vi "pid-tuning.vi"() -> ()   [LabVIEW 2019]
uses:
  <vilib>/DAQmx/read.llb/DAQmx Read (Analog 1D DBL 1Chan NSamp).vi
  <vilib>/Analysis/baseanly.llb/Mean (DBL).vi
  <vilib>/DAQmx/write.llb/DAQmx Write (Analog DBL 1Chan 1Samp).vi
  <vilib>/DAQmx/create/channels.llb/DAQmx Create Channel (AO-Current-Basic).vi
  <vilib>/DAQmx/create/channels.llb/DAQmx Create Channel (AI-Current-Basic).vi
  <vilib>/DAQmx/miscellaneous.llb/DAQmx Fill In Error Info.vi
  <vilib>/addons/control/pid/pid.llb/PID (DBL).vi
  <vilib>/Analysis/NI_AALBase.lvlib
  <vilib>/addons/control/pid/NI_PID_pid.lvlib
panel:
  out "PID FINAL POWER":dbl
  in  "stop":bool
  out "PID START TIME":dbl
  in  "Tabs":T1(tab)
  in  "POWER CONTROL":dbl format="%#_13g"
  in  "ENABLE FURNACE TEST":bool[](array[boolean])=[FALSE]
  in  "STOP FURNACE TEST":bool[](array[boolean])=[FALSE]
  out "PYROMETER READING":dbl
  in  "RAMP UP POWER":dbl format="%#_13g"
  out "TEMPERATURE OVER TIME":cluster{dbl[], dbl[]}[](graph)
  out "CURRENT TEMPERATURE (C)":dbl
  in  "PID SETPOINT":dbl=820.0
  in  "Clear Data":bool
  in  "Restart PID":bool
  in  "PID gains":T2={"proportional gain (Kc)"=5e-05, "integral time (Ti, min)"=1.5, "derivative time (Td, min)"=0.0} {"derivative time (Td, min)" format="%.8f"; "integral time (Ti, min)" format="%.24f"; "proportional gain (Kc)" format="%.8f"}
  out "POWER LEVEL OUTPUT (%)":dbl
  in  "Time Target (s)":dbl=1.0
  in  "Auto Ramp":bool
  out "Current setpoint":dbl
  in  "Max temp":dbl
  out "Time has Elapsed 2":bool caption="Time has Elapsed"
  out "CURRENT RAMP DOWN POWER LEVEL":string
  out "PYROMETER READING 2":dbl
  in  "RAMP DOWN TIME (min)":dbl=10.0
  in  "Mode":T3(ring)
  out "PYROMETER TEMP":dbl
  in  "POWER OUT":dbl format="%#_13g"
  in  "STOP FURNACE":bool[](array[boolean])
  in  "ENABLE FURNACE":bool[](array[boolean])
  out "DONE":bool
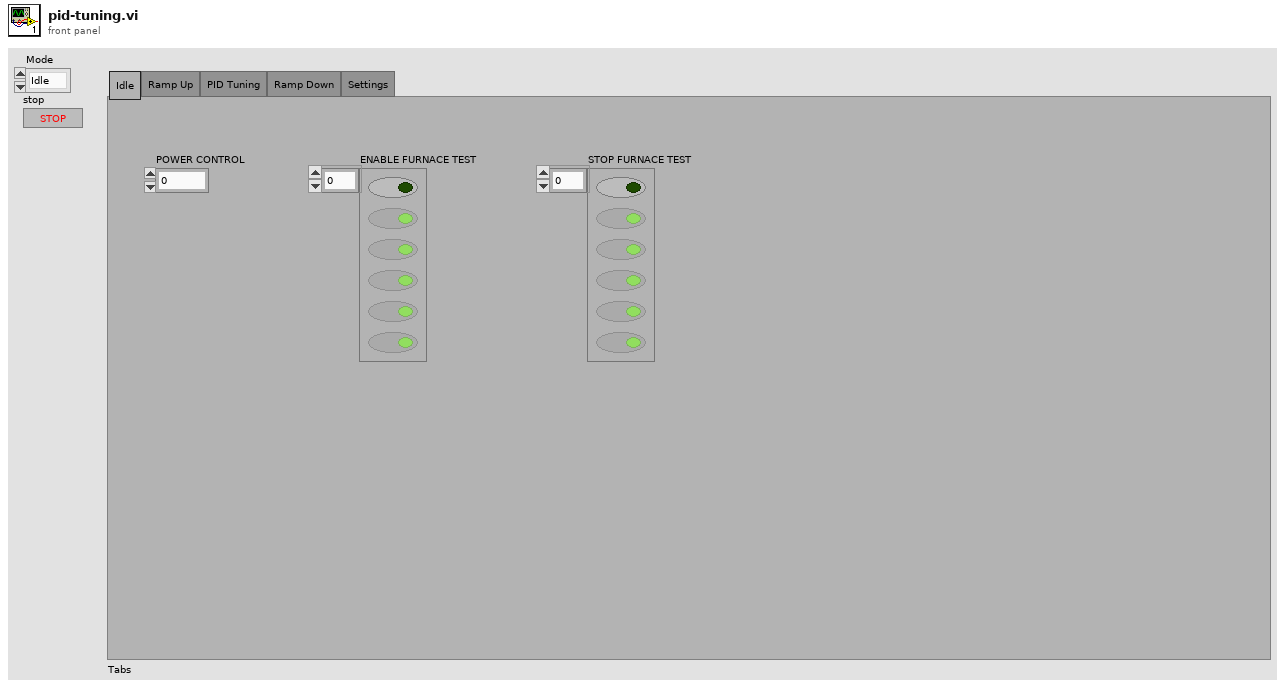
[diagram p1: front panel]
types:
  T1 = enum32{"Idle", "Ramp Up", "PID Tuning", "Ramp Down", "Settings"}
  T2 = cluster{"proportional gain (Kc)":dbl, "integral time (Ti, min)":dbl, "derivative time (Td, min)":dbl}
  T3 = enum16{"Idle", "Ramp Up", "PID Tune", "Ramp Down"}
  T4 = enum8{"Enabled", "Disabled", "Disabled and Grayed Out"}
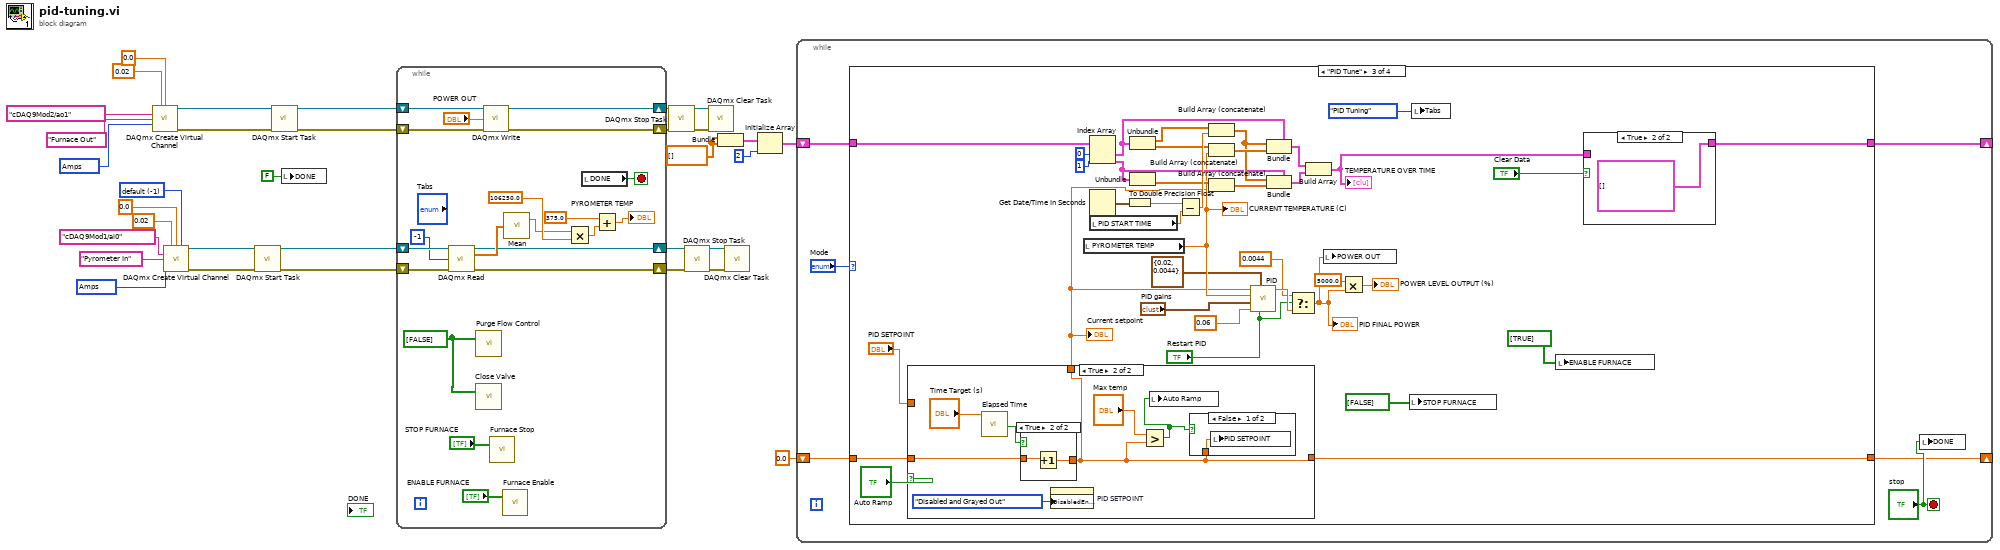
[diagram p0: block diagram]
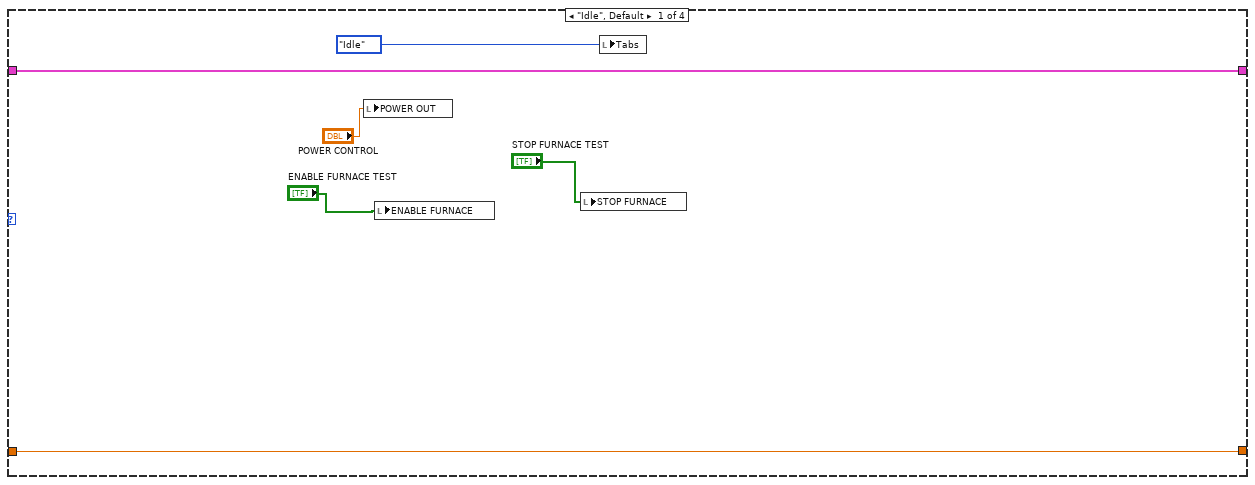
[diagram p2: hidden frame]
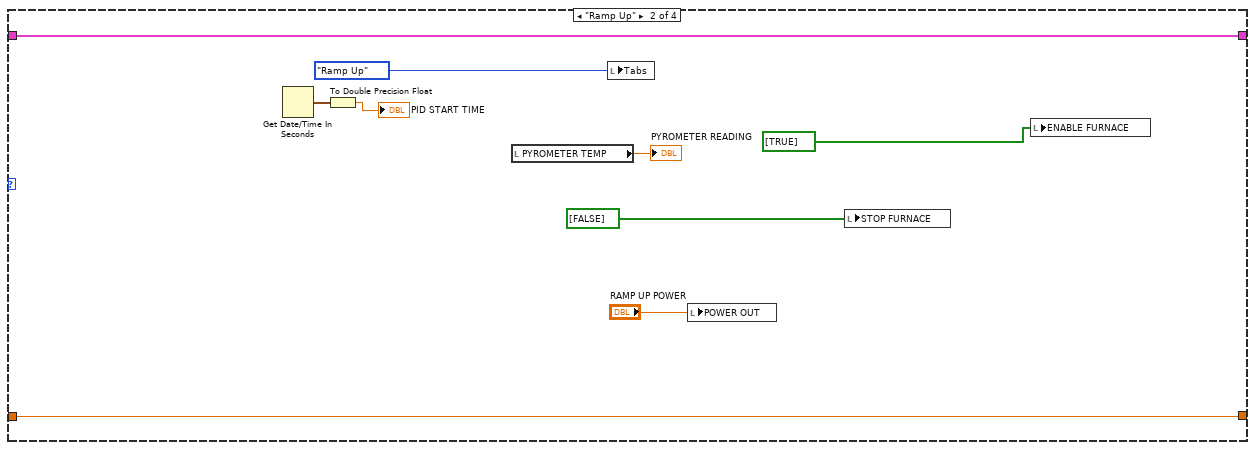
[diagram p3: hidden frame]
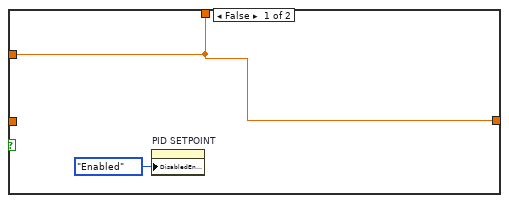
[diagram p4: hidden frame]
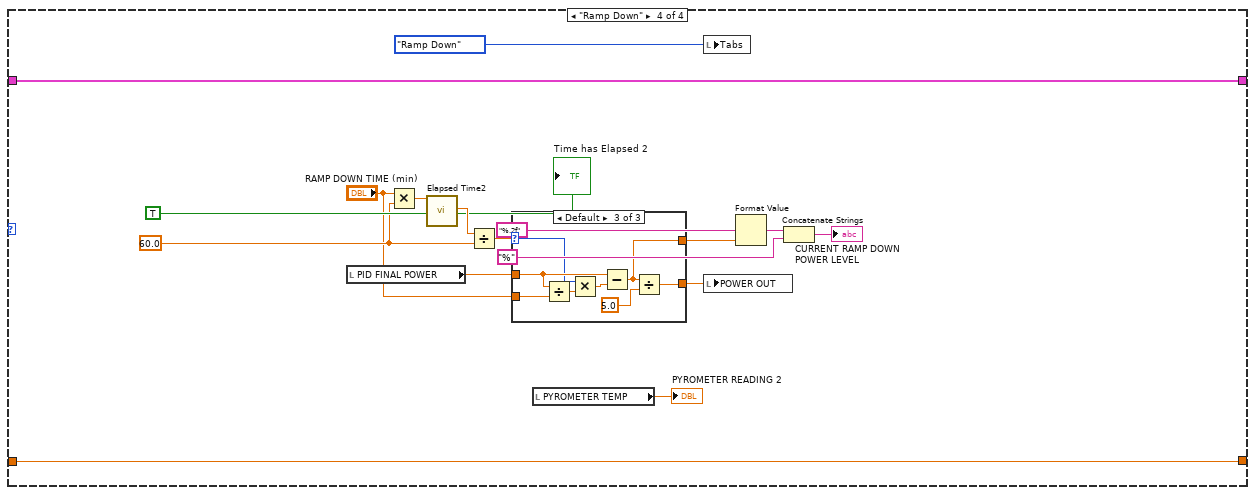
[diagram p8: hidden frame]
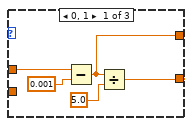
[diagram p9: hidden frame]
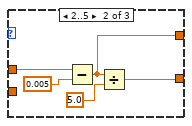
[diagram p10: hidden frame]
diagram:
  w10 = -1 items=["default"=-1, "RSE"=10083, "NRSE"=10078, "Differential"=10106, "Pseudodifferential"=12529] ("input terminal configuration")
  w11 = 10342 items=["Amps"=10342, "From Custom Scale"=10065] ("units")
  w27 = 10342 items=["Amps"=10342, "From Custom Scale"=10065] ("units")
  w32 = dbl[] []
  n1 = call-poly <vilib>:"DAQmx Create Virtual Channel.vi"("maximum value"=0.02, "minimum value"=0.0, "physical channels"=tag "cDAQ9Mod2/ao1", "name to assign"="Furnace Out", "units"=w27) -> ("task out"=w18:refnum<k21>, "error out"=w17:errorcluster)  [unwired: 9 in]
  n2 = call-poly <vilib>:"DAQmx Create Virtual Channel.vi"("maximum value"=0.02, "minimum value"=0.0, "input terminal configuration"=w10, "physical channels"=tag "cDAQ9Mod1/ai0", "name to assign"="Pyrometer In", "units"=w11) -> ("task out"=w9:refnum<k21>, "error out"=w8:errorcluster)  [unwired: 8 in]
  n3 = call <vilib>:"DAQmx Start Task.vi"("task/channels in"=w9, "error in"=w8) -> ("task out"=w7:refnum<k21>, "error out"=w6:errorcluster)  [unwired: 12 in]
  n4 = call <vilib>:"DAQmx Start Task.vi"("task/channels in"=w18, "error in"=w17) -> ("task out"=w20:refnum<k21>, "error out"=w19:errorcluster)  [unwired: 12 in]
  n5 = local write "DONE"(FALSE ("DONE")) -> ()
  n6 = while {
    shift-right: [w43] -> w24
    shift-left: w20 -> [w46]
    shift-right: [w42] -> w23
    shift-left: w19 -> [w45]
    shift-right: [w35] -> w4
    shift-left: w7 -> [w39]
    shift-right: [w34] -> w3
    shift-left: w6 -> [w37]
    stop <- w53 stop-if-true
    w47 = bool[] [FALSE] ("data")
    n7 = call-poly <vilib>:"DAQmx Read.vi"("task/channels in"=w39, "number of samples per channel"=-1, "error in"=w37) -> ("task out"=w35:refnum<k21>, "data"=w36:dbl[], "error out"=w34:errorcluster)  [unwired: 10 in]
    n8 = call "Purge Flow Control"("data"=w47) -> ()  [unwired: 17 in, 2 out]
    n9 = call "Close Valve"("data"=w47) -> ()  [unwired: 17 in, 2 out]
    n10 = call-poly <vilib>:"DAQmx Write.vi"("task/channels in"=w46, "data"="POWER OUT", "error in"=w45) -> ("task out"=w43:refnum<k21>, "error out"=w42:errorcluster)  [unwired: 10 in, 1 out]
    n11 = call "Furnace Stop"("data"="STOP FURNACE") -> ()  [unwired: 17 in, 2 out]
    n12 = call "Furnace Enable"("data"="ENABLE FURNACE") -> ()  [unwired: 17 in, 2 out]
    n13 = call-poly <vilib>:"Mean.vi"("X"=w36) -> ("mean"=w40:dbl)  [unwired: 1 out]
    n14 = Multiply(x=w40, y=106250.0) -> (x*y=w49:dbl)
    n15 = local read "DONE"() -> (w53:bool)
    n16 = Add(x=375.0, y=w49) -> (x+y=→"PYROMETER TEMP":dbl)
  }
  n17 = call <vilib>:"DAQmx Stop Task.vi"("task/channels in"=w24, "error in"=w23) -> ("task out"=w22:refnum<k21>, "error out"=w21:errorcluster)  [unwired: 12 in]
  n18 = call <vilib>:"DAQmx Stop Task.vi"("task/channels in"=w4, "error in"=w3) -> ("task out"=w5:refnum<k21>, "error out"=w2:errorcluster)  [unwired: 12 in]
  n19 = call <vilib>:"DAQmx Clear Task.vi"("task in"=w22, "error in"=w21) -> ()  [unwired: 13 in, 1 out]
  n20 = Bundle(w32, w32) -> (w33:cluster{dbl[], dbl[]})  [unwired: 1 in]
  n21 = call <vilib>:"DAQmx Clear Task.vi"("task in"=w5, "error in"=w2) -> ()  [unwired: 13 in, 1 out]
  n22 = Initialize Array(w33, 2 ("dimension size")) -> (w30:cluster{dbl[], dbl[]}[])
  n23 = while {
    shift-right: [w57] -> _
    shift-left: w30 -> [w58]
    shift-right: [w55] -> _
    shift-left: 0.0 ("PID SETPOINT") -> [w54]
    stop <- "stop" stop-if-true
    n24 = case shown="\"PID Tune\"" "Mode" {
      tunnel: w58 -> [w64 w70 w96 w132]
      tunnel: [w64 w70 w93 w132] -> w57
      tunnel: [w60 w66 w75 w128] -> w55
      tunnel: w54 -> [w60 w66 w78 w128]
      frame "Idle", Default {
        n25 = local write "POWER OUT"("POWER CONTROL") -> ()
        n26 = local write "ENABLE FURNACE"("ENABLE FURNACE TEST") -> ()
        n27 = local write "STOP FURNACE"("STOP FURNACE TEST") -> ()
        n28 = local write "Tabs"(T1."Idle" ("Tabs")) -> ()
      }
      frame "Ramp Up" {
        n29 = Get Date/Time In Seconds() -> (seconds since 1Jan1904=w69:timestamp)
        n30 = To Double Precision Float(number=w69) -> (double precision float=→"PID START TIME":dbl)
        n31 = local read "PYROMETER TEMP"() -> (→"PYROMETER READING":dbl)
        n32 = local write "Tabs"(T1."Ramp Up" ("Tabs")) -> ()
        n33 = local write "POWER OUT"("RAMP UP POWER") -> ()
        n34 = local write "STOP FURNACE"(bool[] [FALSE] ("ENABLE FURNACE")) -> ()
        n35 = local write "ENABLE FURNACE"(bool[] [TRUE] ("Boolean")) -> ()
      }
      frame "PID Tune" {
        n36 = case shown="True" "Auto Ramp" {
          tunnel: [w113 w115] -> w76
          tunnel: [w113 w115] -> w75
          tunnel: w78 -> [_ w120]
          tunnel: "PID SETPOINT" -> [w113 _]
          frame False {
            n37 = property on="PID SETPOINT" class="DigNum (strict)"("DisabledEnum"=T4."Enabled" ("Disabled")) -> ()  [unwired: 2 in, 2 out]
          }
          frame True {
            n38 = call "Elapsed Time"("Time Target (s)"="Time Target (s)") -> ("Time has Elapsed"=w121:bool)  [unwired: 11 in, 7 out]
            n39 = case shown="True" w121 {
              tunnel: w120 -> [w123 w125]
              tunnel: [w123 w124] -> w115
              frame False {
              }
              frame True {
                n40 = Increment(x=w125) -> (x+1=w124:dbl)
              }
            }
            n41 = property on="PID SETPOINT" class="DigNum (strict)"("DisabledEnum"=T4."Disabled and Grayed Out" ("Disabled")) -> ()  [unwired: 2 in, 2 out]
            n42 = Greater?(x="Max temp", y=w115) -> (0:w116:bool)
            n43 = local write "Auto Ramp"(w116) -> ()
            n44 = case shown="False" w116 {
              tunnel: w115 -> [w122 _]
              frame False {
                n45 = local write "PID SETPOINT"(w122) -> ()
              }
              frame True {
              }
            }
          }
        }
        "Current setpoint" <- w76
        n46 = local read "PYROMETER TEMP"() -> (w85:dbl)
        "CURRENT TEMPERATURE (C)" <- w85
        n47 = Index Array(array=w96, index #1=0 ("index"), index #2=1 ("index")) -> (element #1=w107:cluster{dbl[], dbl[]}, element #2=w99:cluster{dbl[], dbl[]})
        n48 = Get Date/Time In Seconds() -> (seconds since 1Jan1904=w112:timestamp)
        n49 = local read "PID START TIME"() -> (w110:dbl)
        n50 = To Double Precision Float(number=w112) -> (double precision float=w111:dbl)
        n51 = Unbundle(w107) -> (w106:dbl[], w104:dbl[])
        n52 = Unbundle(w99) -> (w103:dbl[])  [unwired: 1 out]
        n53 = Subtract(x=w111, y=w110) -> (x-y=w105:dbl)
        n54 = Build Array (concatenate)(w106, w105) -> (w101:dbl[])
        n55 = Build Array (concatenate)(w104, w85) -> (w102:dbl[])
        n56 = Build Array (concatenate)(w103, w76) -> (w100:dbl[])
        n57 = call-poly <vilib>:"PID.vi"("reinitialize? (F)"="Restart PID", "output range"=cluster{"output high":dbl, "output low":dbl} {"output high"=0.02, "output low"=0.0044}, "dt (s)"=0.06, "PID gains"="PID gains", "process variable"=w85, "setpoint"=w76) -> ("output"=w83:dbl)  [unwired: 4 in, 1 out]
        n58 = Bundle(cluster=w107, w101, w102) -> (w97:cluster{dbl[], dbl[]})
        n59 = Bundle(cluster=w99, w101, w100) -> (w98:cluster{dbl[], dbl[]})
        n60 = Select(t=0.0044, s="Restart PID", f=w83) -> (s? t:f=w80:dbl)
        "PID FINAL POWER" <- w80
        n61 = Build Array(w97, w98) -> (w94:cluster{dbl[], dbl[]}[])
        "TEMPERATURE OVER TIME" <- w94
        n62 = local write "POWER OUT"(w80) -> ()
        n63 = Multiply(x=5000.0 ("y"), y=w80) -> (x*y=→"POWER LEVEL OUTPUT (%)":dbl)
        n64 = local write "STOP FURNACE"(bool[] [FALSE] ("ENABLE FURNACE")) -> ()
        n65 = local write "Tabs"(T1."PID Tuning" ("Tabs")) -> ()
        n66 = local write "ENABLE FURNACE"(bool[] [TRUE] ("Boolean")) -> ()
        n67 = case shown="True" "Clear Data" {
          tunnel: w94 -> [w126 _]
          tunnel: [w126 cluster{dbl[], dbl[]}[] []] -> w93
          frame False {
          }
          frame True {
          }
        }
      }
      frame "Ramp Down" {
        w142 = 60.0 ("y")
        n68 = local read "PID FINAL POWER"() -> (w140:dbl)
        n69 = Multiply(x="RAMP DOWN TIME (min)", y=w142) -> (x*y=w144:dbl)
        n70 = call "Elapsed Time2"("Time Target (s)"=w144, "Auto Reset"=TRUE) -> ("Elapsed Time (s)"=w143:dbl, "Time has Elapsed"=→"Time has Elapsed 2":bool)  [unwired: 10 in, 6 out]
        n71 = Divide(x=w143, y=w142) -> (x/y=w141:dbl)
        n72 = case shown="Default" w141 {
          selector: w141 -> [_ _ w160]
          tunnel: w140 -> [w150 w153 w163]
          tunnel: [w147 w152 w157] -> w139
          tunnel: "RAMP DOWN TIME (min)" -> [_ _ w162]
          tunnel: [w146 w151 w156] -> w134
          frame 0, 1 {
            n73 = Subtract(x=w150, y=0.001) -> (x-y=w146:dbl)
            n74 = Divide(x=w146, y=5.0) -> (x/y=w147:dbl)
          }
          frame 2..5 {
            n75 = Subtract(x=w153, y=0.005) -> (x-y=w151:dbl)
            n76 = Divide(x=w151, y=5.0) -> (x/y=w152:dbl)
          }
          frame Default {
            n77 = Divide(x=w163, y=w162) -> (x/y=w161:dbl)
            n78 = Multiply(x=w160, y=w161) -> (x*y=w159:dbl)
            n79 = Subtract(x=w163, y=w159) -> (x-y=w156:dbl)
            n80 = Divide(x=w156, y=5.0) -> (x/y=w157:dbl)
          }
        }
        n81 = local read "PYROMETER TEMP"() -> (→"PYROMETER READING 2":dbl)
        n82 = local write "Tabs"(T1."Ramp Down" ("Tabs")) -> ()
        n83 = local write "POWER OUT"(w139) -> ()
        n84 = Format Value(format string="%.2f", value (0)=w134) -> (output string=w137:string)  [unwired: 1 in]
        n85 = Concatenate Strings(w137, "%" ("format string")) -> (→"CURRENT RAMP DOWN POWER LEVEL":string)
      }
    }
    n86 = local write "DONE"("stop") -> ()
  }
